vi "BaslineCorrection_04.vi"(9 "Swim Detect Params":T1={"U Thresh"=2.0, "L Thresh"=-2.0, "Driv1 Thresh"=1.0, "Freq Cutoff"=24.0, "STD Scaler"=10.0, "Baseline Freq"=1.2, "Baseline Scaler"=0.95} {"Freq Cutoff" format="%#_13g"; "Driv1 Thresh" format="%#_13g"}, 10 "Sampling Freq":dbl=100.0 format="%#_13g", 11 "Data In":dbl[](array[numeric])) -> (3 "Filtered X":dbl[](array[numeric]))   [LabVIEW 2020]
uses:
  SwimDetectParams.ctl
  <vilib>/Analysis/3filter.llb/Filter Passband Type.ctl
  <vilib>/Analysis/3filter.llb/Zero Phase Filter (DBL).vi
  <vilib>/Analysis/3filter.llb/Butterworth Filter (DBL).vi
  <vilib>/Analysis/NI_AALBase.lvlib
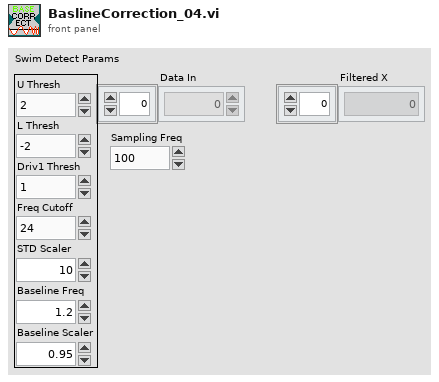
[diagram p1: front panel]
types:
  T1 = typedef "SwimDetectParams.ctl" = cluster{"U Thresh":dbl, "L Thresh":dbl, "Driv1 Thresh":dbl, "Freq Cutoff":dbl, "STD Scaler":dbl, "Baseline Freq":dbl, "Baseline Scaler":dbl}
  T2 = typedef "NI_AALBase.lvlib/Filter Passband Type.ctl" = enum32{"Lowpass", "Highpass", "Bandpass", "Bandstop"}
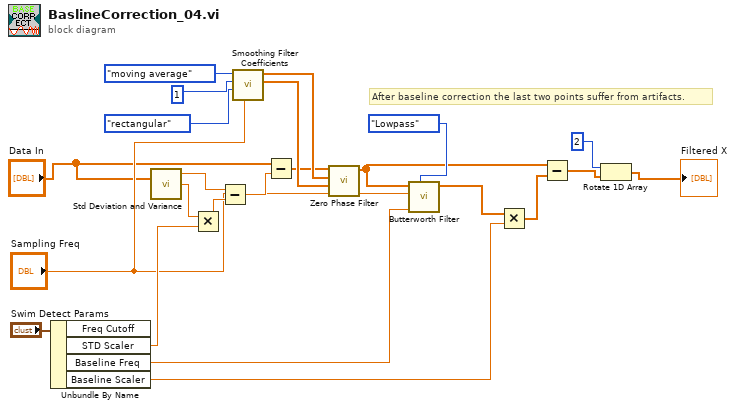
[diagram p0: block diagram]
diagram:
  # "After baseline correction the last two points suffer from artifacts."
  n1 = Unbundle By Name("Swim Detect Params") -> ("STD Scaler"=w18:dbl, "Baseline Freq"=w16:dbl, "Baseline Scaler"=w15:dbl)  [unwired: 1 out]
  n2 = call <vilib>:"Std Deviation and Variance.vi"("X"="Data In") -> ("mean"=w22:dbl, "standard deviation"=w19:dbl)  [unwired: 1 in, 1 out]
  n3 = Multiply(x=w19, y=w18) -> (x*y=w20:dbl)
  n4 = Subtract(x=w22, y=w20) -> (x-y=w21:dbl)
  n5 = call <vilib>:"Smoothing Filter Coefficients.vi"("fs"="Sampling Freq", "shape"=enum16{"rectangular", "triangular"}."rectangular", "half-width"=1, "type"=enum16{"moving average", "exponential"}."moving average") -> ("forward coefficients"=w11:dbl[], "reverse coefficients"=w12:dbl[])  [unwired: 5 in, 1 out]
  n6 = Subtract(x="Data In", y=w21) -> (x-y=w5:dbl[])
  n7 = call-poly <vilib>:"Zero Phase Filter.vi"("Forward Coefficients"=w11, "Reverse Coefficients"=w12, "X"=w5) -> ("Filtered X"=w4:dbl[])  [unwired: 7 in, 1 out]
  n8 = call-poly <vilib>:"Butterworth Filter.vi"("filter type"=Filter_Passband_Type."Lowpass", "low cutoff freq: fl"=w16, "sampling freq: fs"="Sampling Freq", "X"=w4) -> ("Filtered X"=w13:dbl[])  [unwired: 4 in, 1 out]
  n9 = Multiply(x=w13, y=w15) -> (x*y=w14:dbl[])
  n10 = Subtract(x=w4, y=w14) -> (x-y=w2:dbl[])
  n11 = Rotate 1D Array(1:w2, 2:2 ("n")) -> (0:→"Filtered X":dbl[])
